vi "C8855-01_ReadFromSpreadsheetFile.vi"(0 "file path (dialog if empty)":path, 1 "format (%.3f)":string="%.3f", 5 "number of rows (all:-1)":i32=-1, 7 "[pattern]":string caption="[パターン]", 9 "start of read offset (chars.:0 )":i32, 11 "max characters/row  (no limit:0)":i32, 12 "transpose (no:F)":bool, 14 "delimiter (Tab)":string="\t") -> (3 "new file path (Not A Path if cancelled)":path, 4 "all rows":sgl[][](array[numeric]) format="%.3f", 6 "first row":sgl[](array[numeric]) format="%.3f", 10 "mark after read (chars.)":i32, 15 "EOF?":bool)   [LabVIEW 2017]
doc: "Reads a specified number of lines or rows from a numeric text file beginning at a specified character offset and converts the data to a 2D, single-precision array of numbers."
panel:
  in  "type (empty)":sgl[][](array[numeric]) format="%.2f"
  # "row\ncolumn"
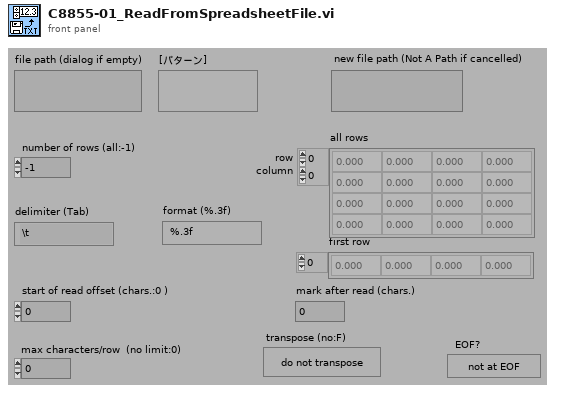
[diagram p1: front panel]
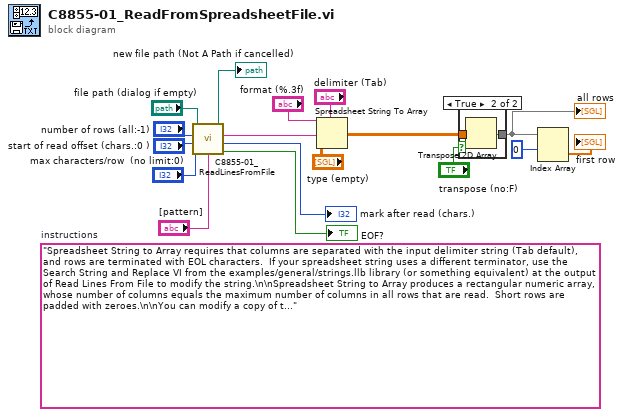
[diagram p0: block diagram]
diagram:
  (unwired) "Spreadsheet String to Array requires that columns are separated with the input delimiter string (Tab default), and rows are terminated with EOL characters.  If your spreadsheet string uses a different terminator, use the Search String and Replace VI from the examples/general/strings.llb library (or something equivalent) at the output of Read Lines From File to modify the string.\n\nSpreadsheet String to Array produces a rectangular numeric array, whose number of columns equals the maximum number of columns in all rows that are read.  Short rows are padded with zeroes.\n\nYou can modify a copy of this VI to return the file contents into arrays of strings by changing all rows, first row, and type (empty) arrays to string arrays and by setting the format to %s."  # instructions
  n1 = call "C8855-01_ReadLinesFromFile.vi"("file path (dialog if empty)"="file path (dialog if empty)", "number of lines (all:-1)"="number of rows (all:-1)", "[pattern]"="[pattern]", "start of read offset (chars.:0 )"="start of read offset (chars.:0 )", "[max characters per line]  (no limit:0)"="max characters/row  (no limit:0)") -> ("new file path (Not A Path if cancelled)"=→"new file path (Not A Path if cancelled)":path, "line string"=w13:string, "mark after read (chars.)"=→"mark after read (chars.)":i32, "EOF?"=→"EOF?":bool)  [unwired: 1 out]
  n2 = Spreadsheet String To Array(delimiter (Tab)="delimiter (Tab)", format string="format (%.3f)", spreadsheet string=w13, array type (2D Dbl)="type (empty)") -> (array=w11:sgl[][])
  n3 = case shown="TRUE" "transpose (no:F)" {
    tunnel: [w18 w20] -> w7
    tunnel: w11 -> [w18 w19]
    frame False {
    }
    frame True {
      n4 = Transpose 2D Array(2D array=w19) -> (transposed array=w20:sgl[][])
    }
  }
  "all rows" <- w7
  n5 = Index Array(array=w7, index (row)=0) -> (element=→"first row":sgl[])  [unwired: 1 in]
